vi "safety_loop.vi"(8 "error in":errorcluster, 11 "Micron config":T1) -> (0 "error out":errorcluster)   [LabVIEW 2014]
uses:
  initialization/micron_config.ctl
  manipulator/squiggle/Host/i2c_interface.ctl
  manipulator/squiggle/Host/fpga_reference.ctl
  Micron params.ctl
  stimulus.ctl
  injection_point.ctl
  filtering/goal_loop_parms.ctl
  mode_conrols.ctl
  manipulator_cal.ctl
  asap/labview/testing/probe_calibration.ctl
  host/network_params.ctl
  cancellation/sq_control_params.ctl
  cancellation/decoupled_gain.ctl
  cancellation/estimation_controls.ctl
  <vilib>/Platform/TimedLoop/XDataNode/timing_clust.ctl
  <vilib>/Platform/TimedLoop/XDataNode/nitl_modes.ctl
  <vilib>/Platform/TimedLoop/XDataNode/wakeup.ctl
  <vilib>/Analysis/baseanly.llb/Real A x B.vi
  <vilib>/Analysis/coordinate.llb/Wrap Angle (array).vi
  <vilib>/Analysis/Matrix/Numeric/Conversions/Array To Matrix - RA2.vi
  initialization/micron_globals.vi
  <vilib>/Platform/TimedLoop/XDataNode/XDataNode.xnode
  <vilib>/Platform/TimedLoop/XDataNode/XDNodeRunTimeDep.lvlib
  <vilib>/Analysis/Matrix/NI_Matrix.lvlib
  <vilib>/Analysis/NI_AALBase.lvlib
  <vilib>/Analysis/NI_AAL_Angle.lvlib
panel:
  in  "Stall time":sgl=500.0
  in  "Compute":bool
  in  "Max rotation (degrees)":dbl[](array[numeric])=[11.088658332824707, 11.088658332824707, 6.0] format="%#.1f"
  out "Angle Out":dbl[](array[numeric]) format="%#.2f"
  # "Parameters:"
  # "The XY angles can be computed from the manipulator calibration, but we don't do that continuously, because one cause of unsafe excursions is the parameters being messed up.  Compute and then make this the default.\nAny Z rotation is unintended, so it should remain small."
  # "Max time that we can be in output saturation before we decide the axis is stalled."
  # "Debug:"
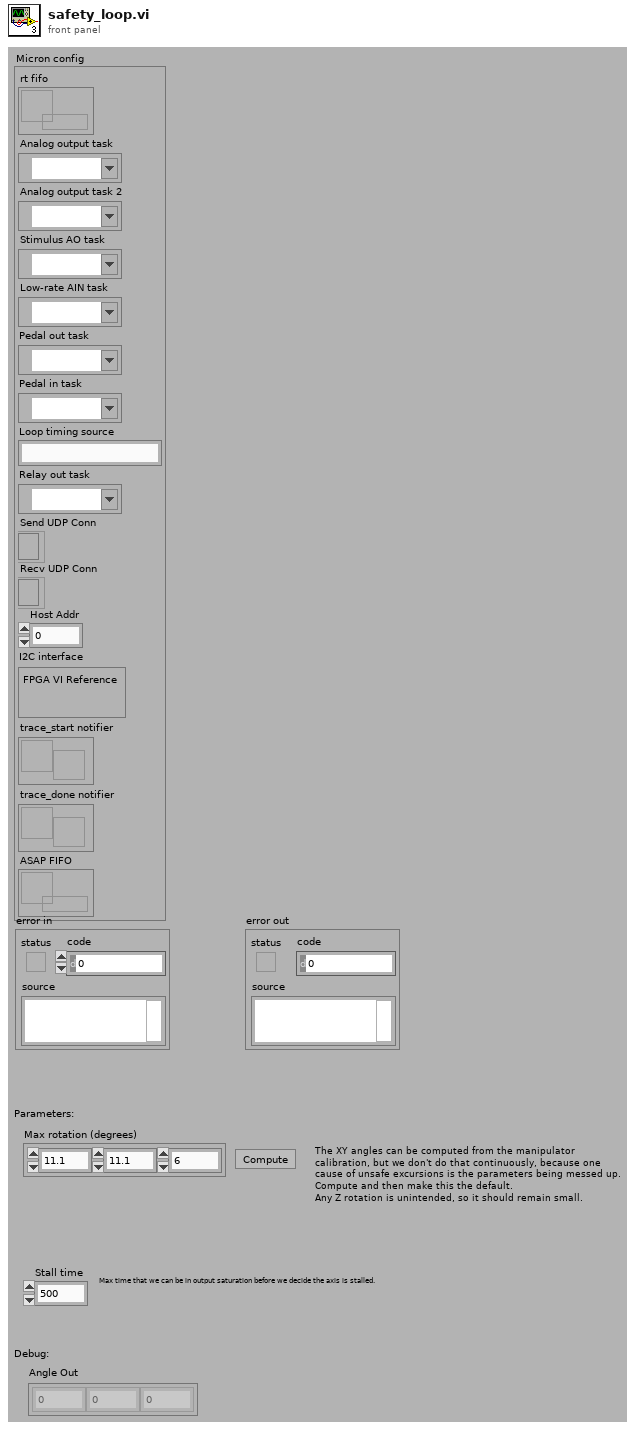
[diagram p1: front panel]
types:
  T1 = typedef "micron_config.ctl" = cluster{"rt fifo":refnum<k33>, "Analog output task":refnum<k21>, "Analog output task 2":refnum<k21>, "Stimulus AO task":refnum<k21>, "Low-rate AIN task":refnum<k21>, "Pedal out task":refnum<k21>, "Pedal in task":refnum<k21>, "Loop timing source":string, "Relay out task":refnum<k21>, "Send UDP Conn":refnum<k16>, "Recv UDP Conn":refnum<k16>, "Host Addr":u32, "I2C interface":T2, "trace_start notifier":refnum<notifier>, "trace_done notifier":refnum<notifier>, "ASAP FIFO":refnum<k33>}
  T2 = typedef "i2c_interface.ctl" = cluster{"FPGA VI Reference":T3}
  T3 = typedef "fpga_reference.ctl" = refnum<k20>
  T4 = typedef "XDNodeRunTimeDep.lvlib/timing_clust.ctl" = cluster{"Expected End [f-1]":u64, "Actual End [f-1]":u64, "Finished Late? [f-1]":bool, "Expected End [i-1]":u64, "Actual End [i-1]":u64, "Finished Late? [i-1]":bool, "Expected Start [i]":u64, "Actual Start [i]":u64, "Expected Start [f]":u64, "Actual Start [f]":u64, "Source Name":string, "Structure Name":string, "Period":i64, "Deadline":i64, "Offset":i64, "Start":i64, "Priority":i32, "Timeout":i32, "Mode":T5, "Wakeup Reason":T6, "Error":errorcluster, "Source Type":string, "Secondary Source Type":string, "Global End Time":u64, "Global Start Time":u64, "Frame Duration":u64, "Iteration Duration":u64, "Assigned CPU":i32, "I/O Scan Engine Mode":u32}
  T5 = typedef "XDNodeRunTimeDep.lvlib/nitl_modes.ctl" = enum32{"No Change", "Process missed periods, maintain original phase", "Discard missed periods, maintain original phase", "Process missed periods, ignore original phase", "Discard missed periods, ignore original phase"}
  T6 = typedef "XDNodeRunTimeDep.lvlib/wakeup.ctl" = enum32{"Normal", "Aborted", "Asynchronous wakeup", "Timing source error", "Timed loop error", "Timeout"}
  T7 = typedef "NI_Matrix.lvlib/RealMatrix.ctl" = dbl[][]
  T8 = typedef "Micron params.ctl" = cluster{"Stimulus":T9, "Goal Filter A":T11, "Mode controls":T12, "Manipulator type":enum16{"Current piezo", "Voltage piezo"}, "Manipulator calibration":T13, "Network":T15, "Goal Filter B":T11, "Cancellation":T16, "Transition time":sgl, "Estimation":T18}
  T9 = typedef "stimulus.ctl" = cluster{"Type":enum16{"Off", "Step", "Sine", "Triangle", "Arbitrary"}, "Phase":dbl, "Amplitude":sgl[], "Injection point":T10, "Closed loop":bool, "Offset":sgl[], "Tip -> world":bool, "Frequency":dbl, "Length":dbl}
  T10 = typedef "injection_point.ctl" = enum16{"Total pose", "V limiter", "Goal ", "Link position", "KF link position", "Inverse kin", "Link goal", "Link error", "Controller", "Output", "Drive", "Light"}
  T11 = typedef "goal_loop_parms.ctl" = cluster{"Speedup max":sgl, "Speedup thresh":sgl, "Speedup nonlin":sgl, "Filters":cluster{"Lower Fc":sgl, "Lower Q":sgl, "Scale factor":sgl, "Upper Fc":sgl, "Upper Q":sgl, "V limit":sgl, "V limit range":sgl}[]}
  T12 = typedef "mode_conrols.ctl" = cluster{"Hold":bool, "Cancellation":bool, "Goal filter":bool, "Trigger":bool}
  T13 = typedef "manipulator_cal.ctl" = cluster{"Tool offsets":sgl[][], "Handle light calibration":T14, "Base pivots":sgl[][], "Output pivots":sgl[][], "Length center":sgl, "Workspace height":sgl[], "Workspace diameter":sgl[], "Stack travel":sgl, "Saturation pos":sgl, "Inverse filters":cluster{"filter structure":enum32{"IIR 2nd Order", "IIR 4th Order"}, "Reverse Coefficients":dbl[], "Forward Coefficients":dbl[]}[], "Strut length":sgl, "Tip light calibration":T14}
  T14 = typedef "probe_calibration.ctl" = sgl[][]
  T15 = typedef "network_params.ctl" = cluster{"Remote Host":string, "Send Status":bool, "Send Port":u16, "Recv Commands":bool, "Recv Port":u16}
  T16 = typedef "sq_control_params.ctl" = cluster{"KP":T17, "KI":sgl, "KD":T17, "Max vel":sgl, "Max acc":sgl, "Int error limit":sgl, "RCM gain":sgl, "Bypass":bool, "Degraded gain":sgl}
  T17 = typedef "decoupled_gain.ctl" = cluster{"XY":sgl, "Rxy":sgl, "Z":sgl, "Rz":sgl}
  T18 = typedef "estimation_controls.ctl" = cluster{"Link":cluster{"Measure noise":dbl[], "Process noise":dbl[], "Alt process noise":dbl[], "Alt turnoff cycles":i32, "Innovation limit":dbl[], "Residue threshold":dbl, "Enable":bool}, "Handle":cluster{"Measure noise":dbl[], "Process noise":dbl[], "State limits":dbl[], "Innovation limit":dbl[], "Prediction Lookahead":sgl, "Enable":bool}}
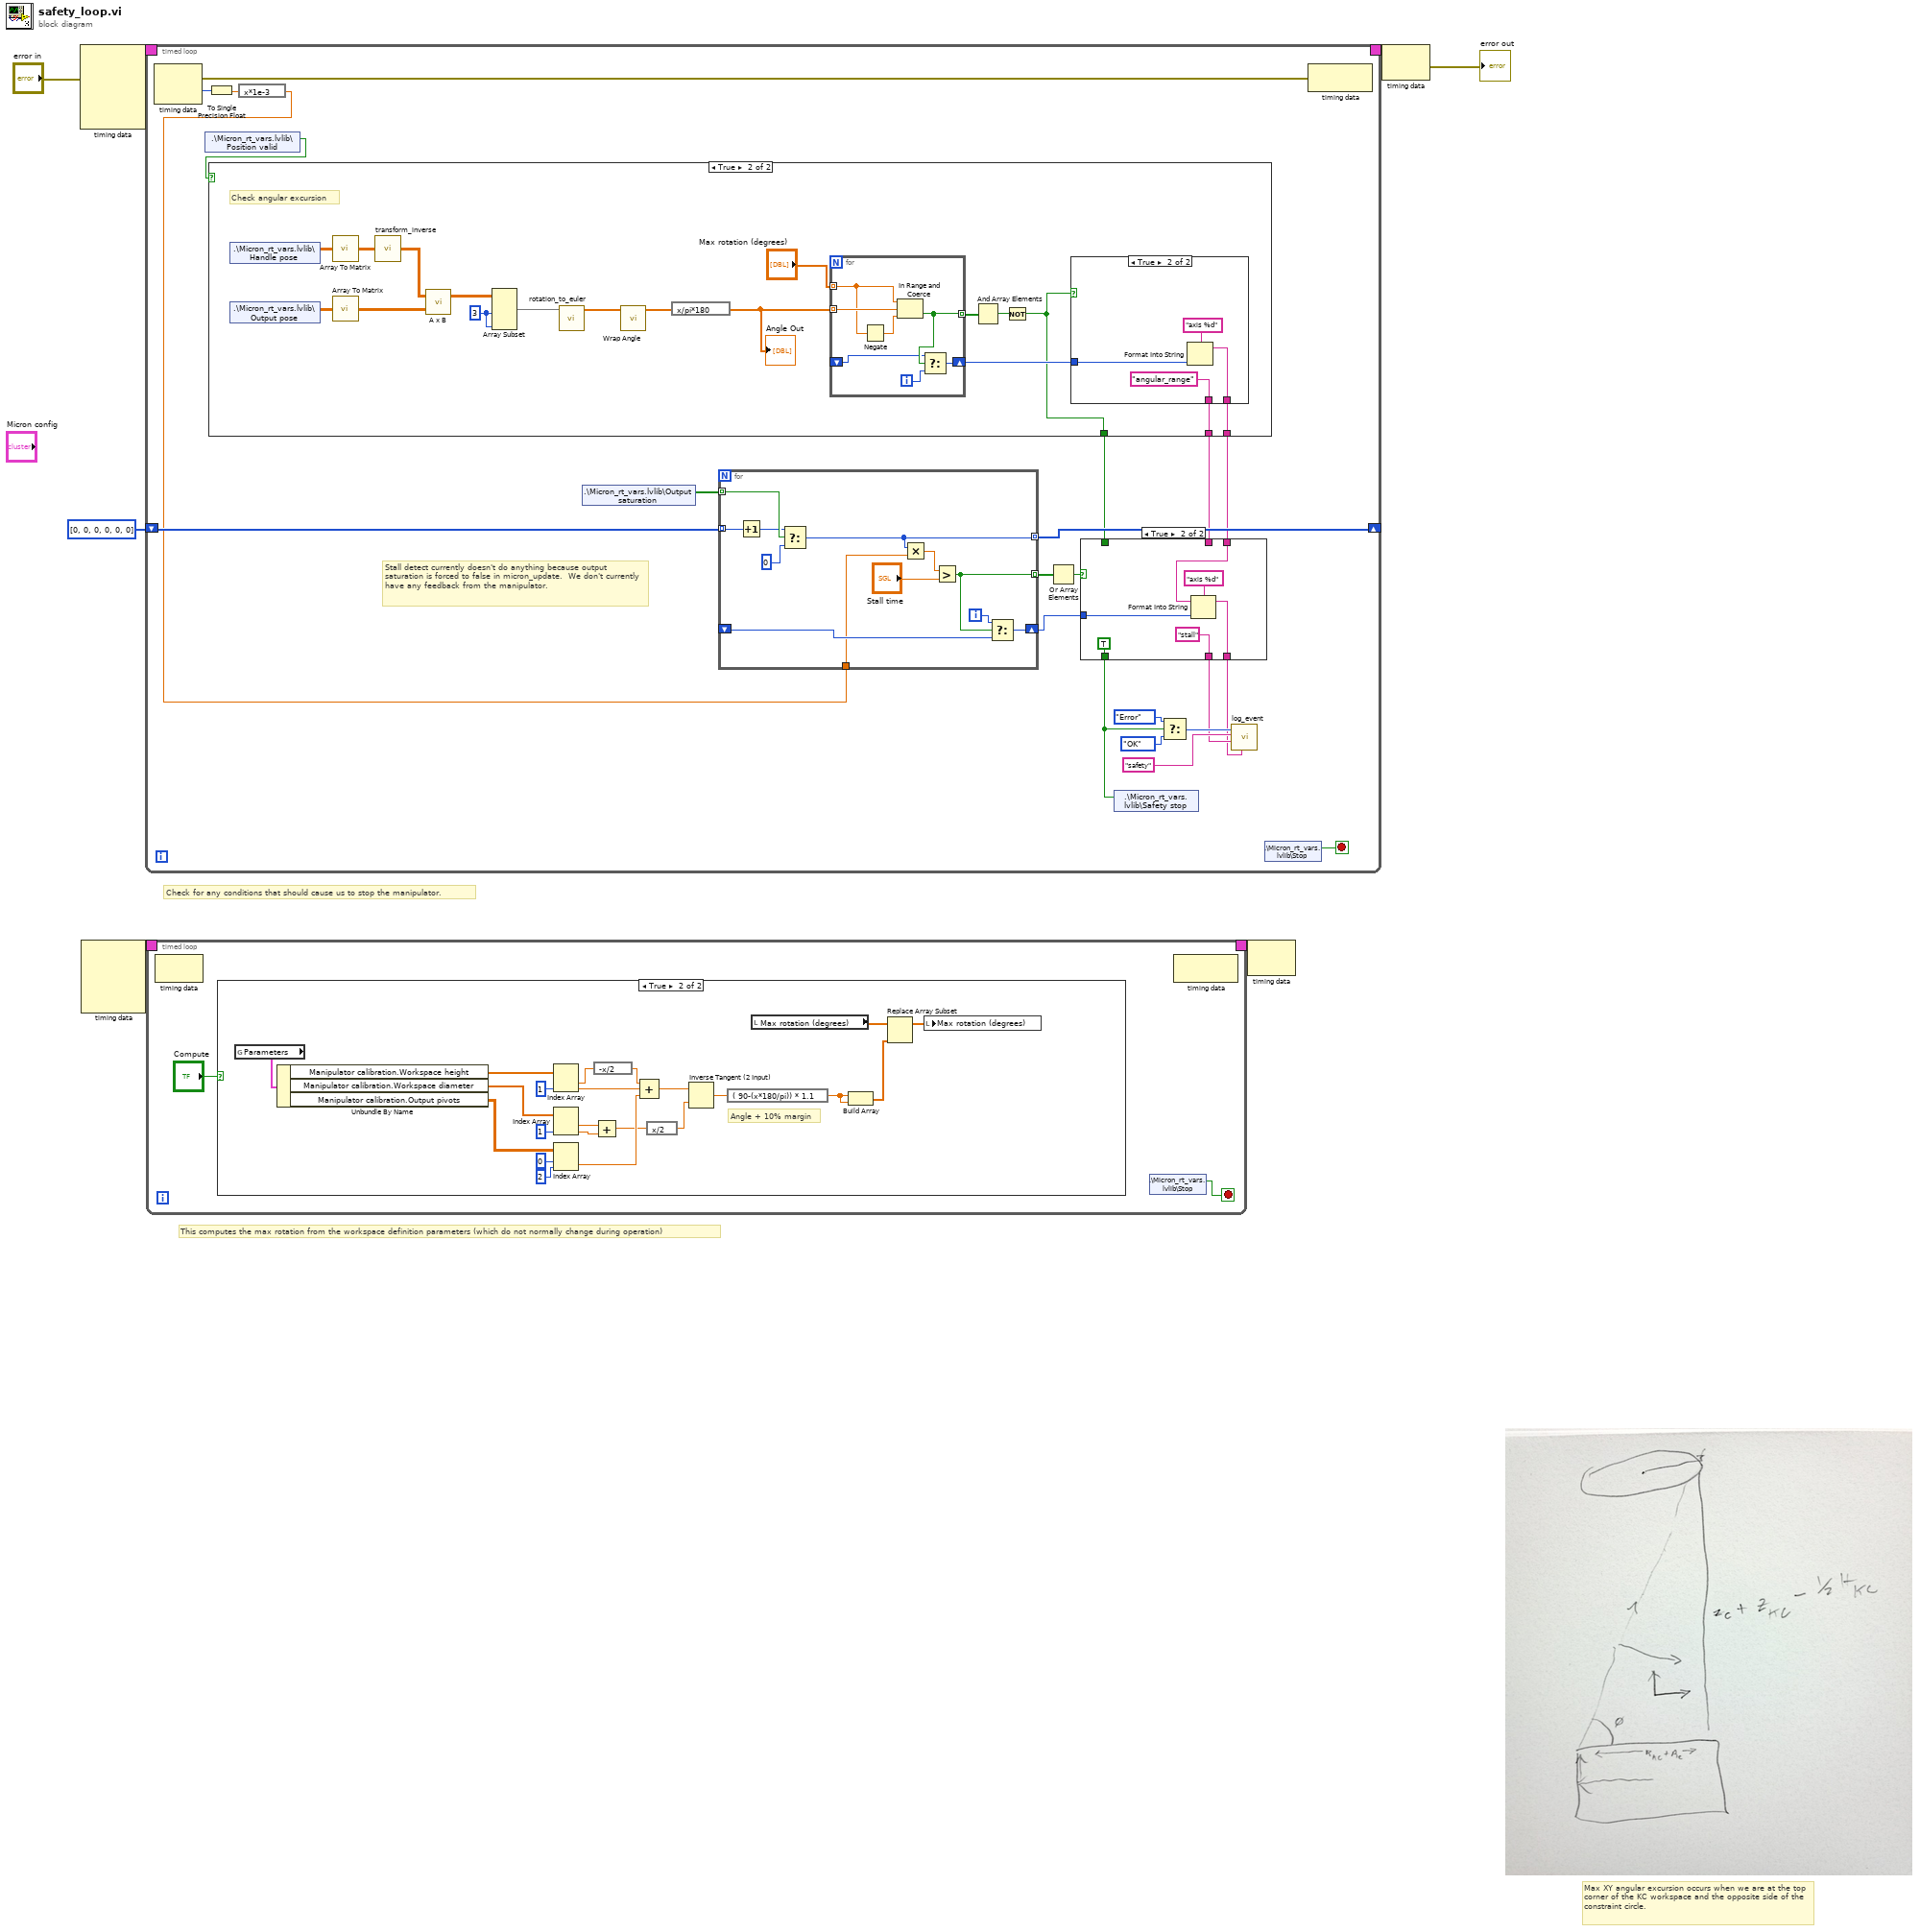
[diagram p0: block diagram]
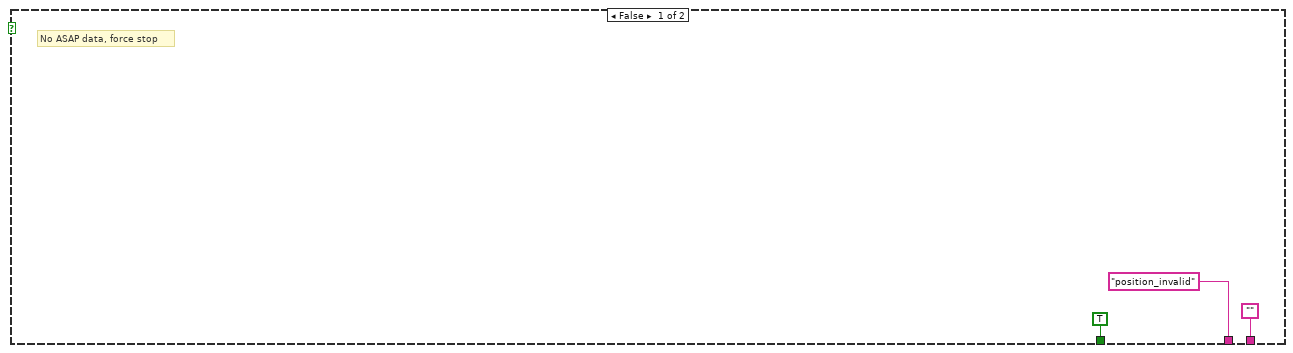
[diagram p4: hidden frame]
diagram:
  # "This computes the max rotation from the workspace definition parameters (which do not normally change during operation)"
  # "Max XY angular excursion occurs when we are at the top corner of the KC workspace and the opposite side of the constraint circle."
  # "Check for any conditions that should cause us to stop the manipulator."
  n1 = node-c288("error in") -> (w7:T4)  [unwired: 1 in, 3 out]
  n2 = node-c288() -> (w4:T4)  [unwired: 4 in]
  n3 = timed-loop {
    timing: w7 -> [_]
    timing-out: [_] -> w6
    shift-right: [w25] -> _
    shift-left: i32[] [0, 0, 0, 0, 0, 0] -> [w26]
    stop <- w29 stop-if-true
    # "Stall detect currently doesn't do anything because output saturation is forced to false in micron_update.  We don't currently have any feedback from the manipulator."
    n4 = node-c288() -> (w28:errorcluster, w21:i64)  [unwired: 1 out]
    n5 = shared-variable ".\\Micron_rt_vars.lvlib\\Position valid"() -> (w11:bool)  [unwired: 2 out]
    n6 = To Single Precision Float(number=w21) -> (single precision float=w20:sgl)
    n7 = case shown="True" w11 {
      tunnel: [TRUE w55] -> w18
      tunnel: ["" w56] -> w17
      tunnel: ["position_invalid" ("format string") w54] -> w16
      frame False {
        # "No ASAP data, force stop"
      }
      frame True {
        w65 = 3 ("length")
        # "Check angular excursion"
        n8 = shared-variable ".\\Micron_rt_vars.lvlib\\Handle pose"() -> (w71:sgl[][])  [unwired: 2 out]
        n9 = shared-variable ".\\Micron_rt_vars.lvlib\\Output pose"() -> (w70:sgl[][])  [unwired: 2 out]
        n10 = call-poly <vilib>:"Array To Matrix.vi"("Real 2D Array"=w71) -> ("Real Matrix"=w69:T7)
        n11 = call-poly <vilib>:"Array To Matrix.vi"("Real 2D Array"=w70) -> ("Real Matrix"=w68:T7)
        n12 = call "transform_inverse.vi"("Transform"=w69) -> ("Inverse transform"=w67:T7)
        n13 = call-poly <vilib>:"A x B.vi"("B"=w68, "A"=w67) -> ("A x B"=w66:T7)  [unwired: 1 out]
        n14 = Array Subset(array=w66, length (row)=w65, length (col)=w65) -> (w64:T7)  [unwired: 2 in]
        n15 = call "rotation_to_euler.vi"("Rotation"=w64) -> ("Theta XYZ"=w61:dbl[])  [unwired: 10 in]
        n16 = call-poly <vilib>:"Wrap Angle.vi"("Angle In"=w61) -> ("Angle Out"=w60:dbl[])  [unwired: 9 in, 1 out]
        n17 = expression code="x/pi*180"(w60) -> (w58:dbl[])
        "Angle Out" <- w58
        n18 = for {
          tunnel: w58 -> [w82] mode=indexing
          tunnel: "Max rotation (degrees)" -> [w80] mode=indexing
          tunnel: [w78] -> w63 mode=indexing
          shift-right: [w79] -> w57
          shift-left: _ -> [w77]
          i -> [w76]
          n19 = Negate(x=w80) -> (-x=w81:dbl)
          n20 = In Range and Coerce(upper limit=w80, x=w82, lower limit=w81) -> (In Range?=w78:bool)  [unwired: 1 out]
          n21 = Select(t=w77, s=w78, f=w76) -> (s? t:f=w79:i32)
        }
        n22 = And Array Elements(Boolean array=w63) -> (logical AND=w62:bool)
        n23 = Not(x=w62) -> (.not. x?=w55:bool)
        n24 = case shown="True" w55 {
          tunnel: w57 -> [_ w75]
          tunnel: [_ w73] -> w56
          tunnel: [_ "angular_range" ("format string")] -> w54
          frame False {
          }
          frame True {
            n25 = Format Into String(format string="axis %d", w75) -> (resulting string=w73:string)  [unwired: 2 in, 1 out]
          }
        }
      }
    }
    n26 = expression code="x*1e-3"(w20) -> (w19:sgl)
    n27 = shared-variable ".\\Micron_rt_vars.lvlib\\Output saturation"() -> (w27:bool[])  [unwired: 1 in, 1 out]
    n28 = for {
      tunnel: w27 -> [w50] mode=indexing
      tunnel: w26 -> [w48] mode=indexing
      tunnel: [w40] -> w25 mode=indexing
      shift-right: [w45] -> w23
      shift-left: _ -> [w43]
      tunnel: [w42] -> w24 mode=indexing
      tunnel: w19 -> [w41]
      i -> [w44]
      n29 = Increment(x=w48) -> (x+1=w47:i32)
      n30 = Select(t=w47, s=w50, f=0) -> (s? t:f=w40:i32)
      n31 = Multiply(x=w40, y=w41) -> (x*y=w39:sgl)
      n32 = Greater?(x=w39, y="Stall time") -> (0:w42:bool)
      n33 = Select(t=w44, s=w42, f=w43) -> (s? t:f=w45:i32)
    }
    n34 = Or Array Elements(Boolean array=w24) -> (logical OR=w22:bool)
    n35 = case shown="True" w22 {
      tunnel: w23 -> [_ w38]
      tunnel: [w31 w36] -> w8
      tunnel: [w32 TRUE] -> w10
      tunnel: w18 -> [w32 _]
      tunnel: w17 -> [w31 w34]
      tunnel: [w30 "stall" ("format string")] -> w9
      tunnel: w16 -> [w30 _]
      frame False {
      }
      frame True {
        n36 = Format Into String(format string="axis %d", initial string=w34, w38) -> (resulting string=w36:string)  [unwired: 1 in, 1 out]
      }
    }
    n37 = shared-variable ".\\Micron_rt_vars.lvlib\\Safety stop"(w10) -> ()  [unwired: 1 in, 1 out]
    n38 = Select(t=enum16{"OK", "Debug", "Warn", "Error"}."Error" ("Severity"), s=w10, f=enum16{"OK", "Debug", "Warn", "Error"}."OK" ("Severity")) -> (s? t:f=w13:enum16{"OK", "Debug", "Warn", "Error"})
    n39 = call "log_event.vi"("Message"=w8, "State"=w9, "Facility"="safety", "Severity"=w13) -> ()  [unwired: 7 in, 1 out]
    n40 = shared-variable ".\\Micron_rt_vars.lvlib\\Stop"() -> (w29:bool)  [unwired: 2 out]
    n41 = node-c288(w28) -> ()  [unwired: 1 out]
  }
  n42 = timed-loop {
    timing: w4 -> [_]
    timing-out: [_] -> w3
    stop <- w89 stop-if-true
    n43 = node-c288() -> ()  [unwired: 1 in, 1 out]
    n44 = case shown="True" "Compute" {
      frame False {
      }
      frame True {
        # "Angle + 10% margin"
        n45 = global read "micron_globals.vi" "Parameters"() -> (w112:T8)
        n46 = Unbundle By Name(w112) -> ("Manipulator calibration.Workspace height"=w108:sgl[], "Manipulator calibration.Workspace diameter"=w111:sgl[], "Manipulator calibration.Output pivots"=w107:sgl[][])
        n47 = Index Array(array=w108, index #2=1 ("index")) -> (element #1=w102:sgl, element #2=w105:sgl)  [unwired: 1 in]
        n48 = Index Array(array=w111, index #2=1 ("index")) -> (element #1=w98:sgl, element #2=w99:sgl)  [unwired: 1 in]
        n49 = Index Array(array=w107, index (row)=0 ("disabled index (row)"), index (col)=2 ("disabled index (col)")) -> (element=w104:sgl)
        n50 = expression code="-x/2"(w102) -> (w101:sgl)
        n51 = Add(x=w98, y=w99) -> (x+y=w96:sgl)
        n52 = Compound Arithmetic op=ADD(w101, w105, w104) -> (w100:sgl)
        n53 = expression code="x/2"(w96) -> (w97:sgl)
        n54 = Inverse Tangent (2 Input)(1:w97, 2:w100) -> (0:w92:sgl)
        n55 = expression code="( 90-(x*180/pi)) * 1.1"(w92) -> (w91:sgl)
        n56 = local read "Max rotation (degrees)"() -> (w95:dbl[])
        n57 = Build Array(w91, w91) -> (w94:sgl[])
        n58 = Replace Array Subset(array=w95, new element=w94) -> (w93:dbl[])  [unwired: 1 in]
        n59 = local write "Max rotation (degrees)"(w93) -> ()
      }
    }
    n60 = shared-variable ".\\Micron_rt_vars.lvlib\\Stop"() -> (w89:bool)  [unwired: 2 out]
    n61 = node-c288() -> ()  [unwired: 1 in, 1 out]
  }
  n62 = node-c288(w3) -> ()  [unwired: 1 out]
  n63 = node-c288(w6) -> (→"error out":errorcluster)
